vi "Set PID values.vi"(8 "D Value":sgl, 9 "I Value":sgl, 10 "P Value":sgl, 11 "Boolean":bool) -> ()   [LabVIEW 2012]
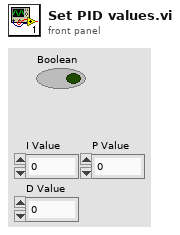
[diagram p1: front panel]
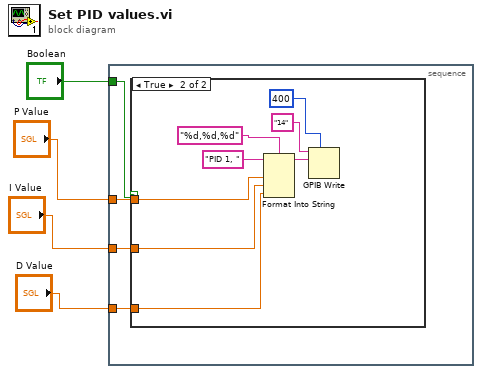
[diagram p0: block diagram]
diagram:
  n1 = stacked-sequence {
    tunnel: "D Value" -> [w8]
    tunnel: "I Value" -> [w7]
    tunnel: "P Value" -> [w6]
    tunnel: "Boolean" -> [w5]
    frame #0 {
      n2 = case shown="True" w5 {
        tunnel: w8 -> [_ w11]
        tunnel: w7 -> [_ w10]
        tunnel: w6 -> [_ w9]
        frame False {
        }
        frame True {
          n3 = Format Into String(format string="%d,%d,%d", initial string="PID 1, ", w9, w10, w11) -> (resulting string=w16:string)  [unwired: 1 in, 1 out]
          n4 = GPIB Write(0:"14", 1:w16, 4:400) -> ()  [unwired: 2 in, 2 out]
        }
      }
    }
  }
